vi "CheesyEagle Receiver.vi"() -> ()   [LabVIEW 2013]
uses:
  <vilib>/Utility/error.llb/DialogType.ctl
panel:
  out "data out":string
  in  "stop":bool
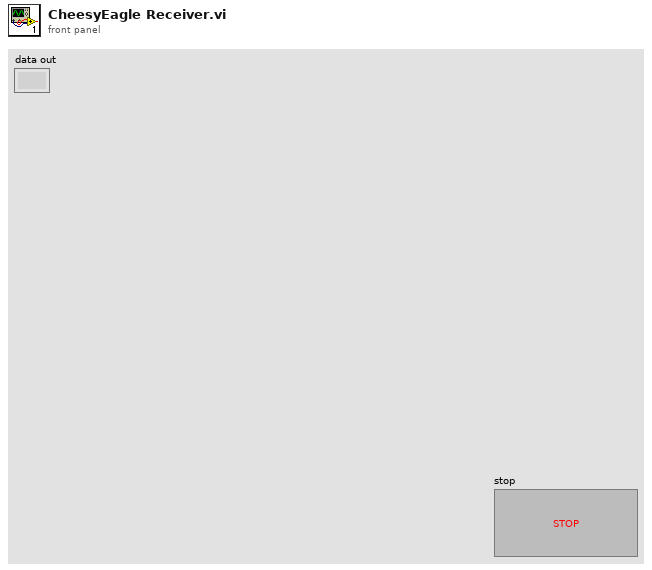
[diagram p1: front panel]
types:
  T1 = typedef "DialogType.ctl" = u16
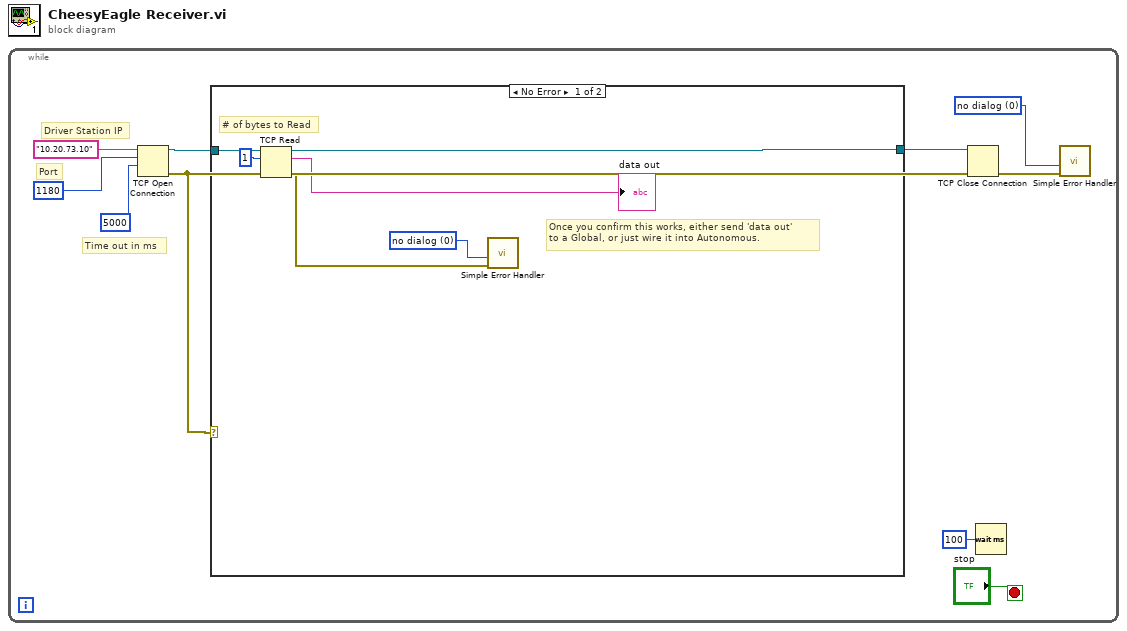
[diagram p0: block diagram]
diagram:
  n1 = while {
    stop <- "stop" stop-if-true
    w1 = T1 0 items=["no dialog", "OK message", "continue or stop message", "OK message + warnings", "continue/stop + warnings"] ("type of dialog (OK msg:1)")
    # "Time out in ms"
    # "Port"
    # "Driver Station IP"
    n2 = TCP Open Connection(address="10.20.73.10", remote port or service name=u16 1180, timeout ms (60000)=5000) -> (connection ID=w6:refnum<k5>, error out=w3:errorcluster)  [unwired: 2 in]
    n3 = case shown="No Error" w3 {
      tunnel: w6 -> [w16 w17]
      tunnel: [w13 w17] -> w4
      frame No Error {
        w11 = T1 0 items=["no dialog", "OK message", "continue or stop message", "OK message + warnings", "continue/stop + warnings"] ("type of dialog (OK msg:1)")
        # "Once you confirm this works, either send 'data out'\nto a Global, or just wire it into Autonomous."
        # "# of bytes to Read"
        n4 = TCP Read(connection ID=w16, bytes to read=1) -> (connection ID out=w13:refnum<k5>, data out=→"data out":string, error out=w12:errorcluster)  [unwired: 3 in]
        n5 = call <vilib>:"Simple Error Handler.vi"("type of dialog (OK msg:1)"=w11, "error in (no error)"=w12) -> ()  [unwired: 3 in, 5 out]
      }
      frame Error {
      }
    }
    n6 = TCP Close Connection(connection ID=w4, error in (no error)=w3) -> (error out=w2:errorcluster)  [unwired: 1 in, 1 out]
    n7 = Wait (ms)(milliseconds to wait=u32 100) -> ()  [unwired: 1 out]
    n8 = call <vilib>:"Simple Error Handler.vi"("type of dialog (OK msg:1)"=w1, "error in (no error)"=w2) -> ()  [unwired: 3 in, 5 out]
  }
